vi "MAC END.vi"(0 "System no.":i32=1 min=1 max=4 step=1, 5 "error in":errorcluster) -> (19 "error out":errorcluster)   [LabVIEW 2020]
doc: "Stops current macro recording.\n\nE-516: Macro will not be saved to FLASH until WPA.vi was run. Changes not saved with WPA are only present in RAM and will be lost when the controller is powered off.\n\nE-816: Macro will not be saved to FLASH until WPA .vi was run. Changes not saved with WPA are only present in RAM and will be lost when the controller is powered off. This command cannot be issued to a slave. Check controller manual to find out if MAC END is supported.\n\nM-8X0: Only for GCS syntax version = GCS 2.0 or higher (check with CSV?.vi. If CSV?.vi is not supported, syntax version is GCS 1.0)."
panel:
  # "Stops current macro recording."
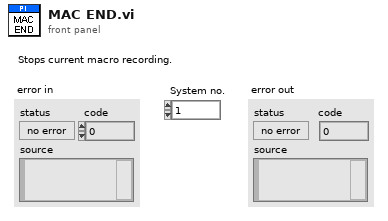
[diagram p1: front panel]
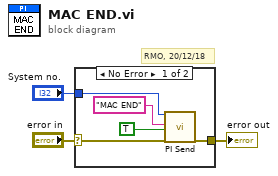
[diagram p0: block diagram]
diagram:
  # "RMO, 20/12/18"
  n1 = case shown="No Error" "error in" {
    selector: "error in" -> [w4 w9]
    tunnel: "System no." -> [w6 _]
    tunnel: [w5 w9] -> w2
    frame No Error {
      n2 = call "PI Send.vi"("System no."=w6, "String to send"="MAC END", "Attach termination char.?"=TRUE ("Attach Linefeed?"), "error in"=w4) -> ("error out"=w5:errorcluster)  [unwired: 2 in, 13 out]
    }
    frame Error {
    }
  }
  "error out" <- w2
